vi "Write ARN.vi"(8 "error in (no error)":errorcluster, 10 "Amazon Resource Name":string, 11 "ARN":refnum<class "ARN.lvclass">) -> (0 "error out":errorcluster, 3 "ARN out":refnum<class "ARN.lvclass">)   [LabVIEW 2015, in "NI_AWS_Core.lvlib" / "ARN.lvclass"]
uses:
  ARN.lvclass
  ARN.lvclass/ARN.ctl
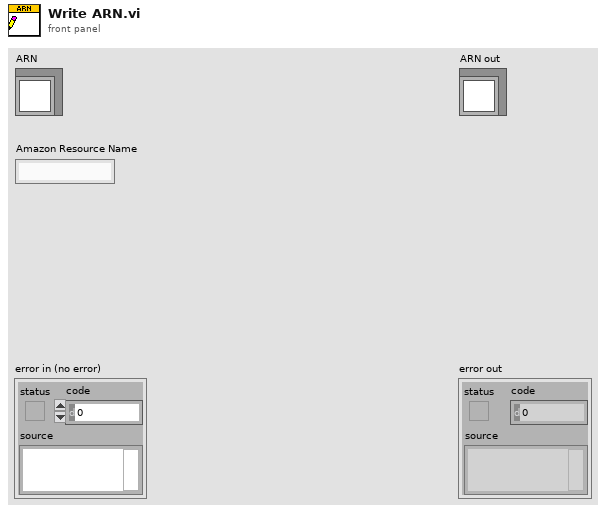
[diagram p1: front panel]
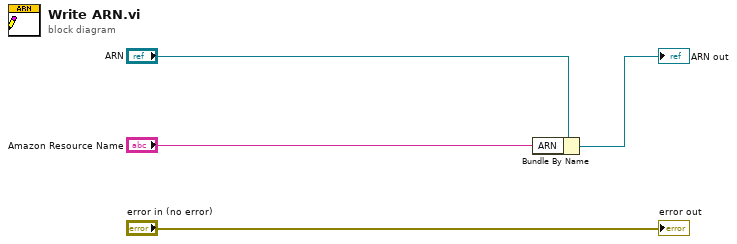
[diagram p0: block diagram]
diagram:
  n1 = Bundle By Name(cluster="ARN", "ARN"="Amazon Resource Name") -> (→"ARN out":refnum<class "ARN.lvclass">)
  "error out" <- "error in (no error)"
